vi "calculator.vi"() -> ()   [LabVIEW 2020]
panel:
  out "Numeric 3":dbl
  in  "Numeric 2":dbl
  in  "Numeric":dbl
  in  "Enum":enum16{"Add", "Sub", "Mul", "Div"}(ring)
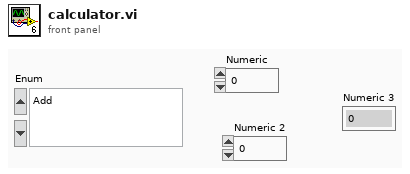
[diagram p1: front panel]
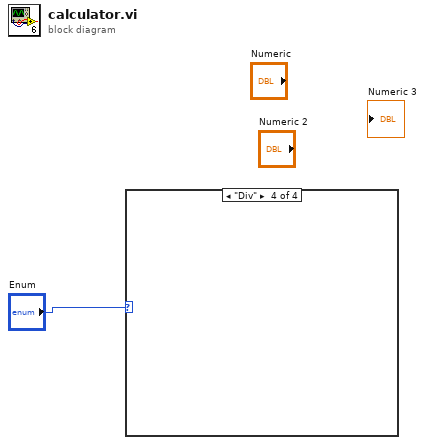
[diagram p0: block diagram]
diagram:
  n1 = case shown="\"Div\"" "Enum" {
    frame "Add", Default {
    }
    frame "Sub" {
    }
    frame "Mul" {
    }
    frame "Div" {
    }
  }
